vi "Get Temperature in Celsius.vi"(8 "error in":errorcluster, 11 "PPT in":refnum<class "PPT.lvclass">) -> (0 "error out":errorcluster, 2 "Temperature":dbl, 3 "PPT out":refnum<class "PPT.lvclass">)   [LabVIEW 2014, in "PPT Library.lvlib" / "PPT.lvclass"]
doc: "Set the transceiver operating parameters. See PPT documentation to determine how the input parameter is applied."
uses:
  PPT.lvclass
  reusable/Session APIs/Serial/Serial Session.lvclass
  PPT.lvclass/PPT.ctl
  reusable/Session APIs/Serial/Public/Asynchronous Write.vi
  reusable/Session APIs/Serial/Public/Asynchronous Read.vi
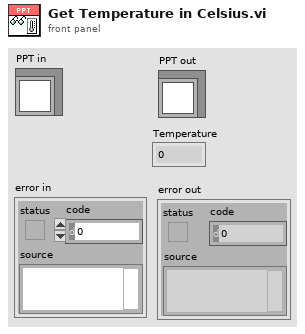
[diagram p1: front panel]
types:
  T1 = typedef "Session - Root.lvclass/Session Handle.ctl" = refnum<data-value>
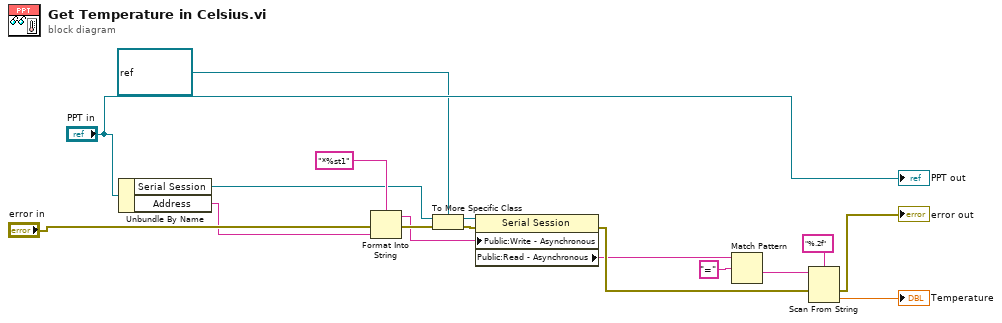
[diagram p0: block diagram]
diagram:
  n1 = Unbundle By Name("PPT in") -> ("Serial Session"=w2:T1, "Address"=w1:string)
  n2 = Format Into String(format string="*%st1", error in="error in", w1) -> (resulting string=w4:string, error out=w5:errorcluster)  [unwired: 1 in]
  n3 = To More Specific Class(target class=refnum<data-value> refnum ("Serial Session"), reference=w2, error in=w5) -> (specific class reference=w8:refnum<data-value>, error out=w7:errorcluster)
  n4 = property class="Serial Session"(reference=w8, error in=w7, "Public:Write - Asynchronous"=w4) -> (error out=w13:errorcluster, "Public:Read - Asynchronous"=w12:string)  [unwired: 1 out]
  n5 = Match Pattern(string=w12, regular expression="=") -> (after substring=w10:string)  [unwired: 1 in, 3 out]
  n6 = Scan From String(format string="%.2f", input string=w10, error in=w13) -> (error out=→"error out":errorcluster, output 1=→"Temperature":dbl)  [unwired: 2 in, 2 out]
  "PPT out" <- "PPT in"
